vi "BoundAngle0To360.vi"(1 "angle":dbl) -> (0 "bound angle":dbl)   [LabVIEW 2015]
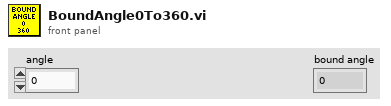
[diagram p1: front panel]
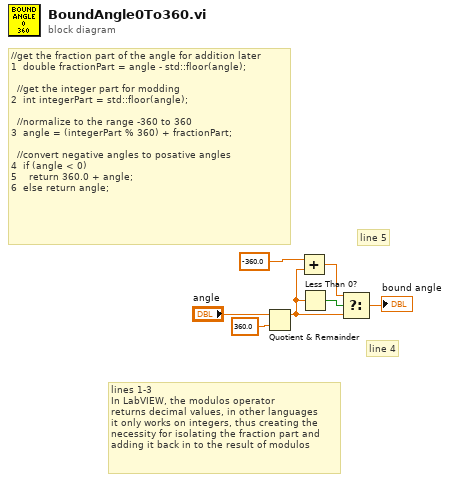
[diagram p0: block diagram]
diagram:
  # "line 4"
  # "line 5"
  # "lines 1-3\nIn LabVIEW, the modulos operator\nreturns decimal values, in other languages\nit only works on integers, thus creating the\nnecessity for isolating the fraction part and \nadding it back in to the result of modulos"
  # "//get the fraction part of the angle for addition later\n1  double fractionPart = angle - std::floor(angle);\n\n  //get the integer part for modding\n2  int integerPart = std::floor(angle);\n\n  //normalize to the range -360 to 360\n3  angle = (integerPart % 360) + fractionPart;\n\n  //convert negative angles to posative angles\n4  if (angle < 0)\n5    return 360.0 + angle;\n6  else return angle;"
  n1 = Quotient & Remainder(x="angle", y=360.0) -> (x-y*floor(x/y)=w2:dbl)  [unwired: 1 out]
  n2 = Add(x=-360.0, y=w2) -> (x+y=w3:dbl)
  n3 = Less Than 0?(x=w2) -> (x < 0?=w5:bool)
  n4 = Select(t=w3, s=w5, f=w2) -> (s? t:f=→"bound angle":dbl)
